vi "GetMeanCurrent.vi"(8 "error in (no error)":errorcluster, 11 "TecellaChannel in":refnum<class "TecellaChannel.lvclass">) -> (0 "error out":errorcluster, 2 "Mean Current (nA)":dbl, 3 "TecellaChannel out":refnum<class "TecellaChannel.lvclass">)   [LabVIEW 2009, in "TecellaChannel.lvclass"]
uses:
  TecellaChannel.lvclass
  TecellaChannel.lvclass/TecellaChannel.ctl
  TecellaClient/TecellaClient.lvclass
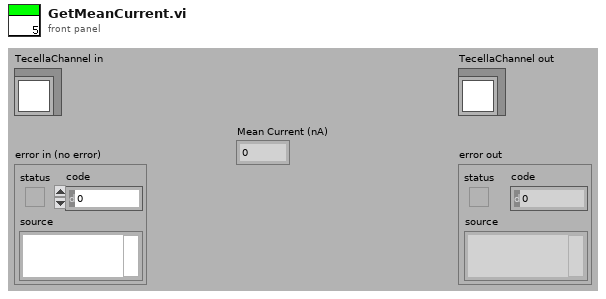
[diagram p1: front panel]
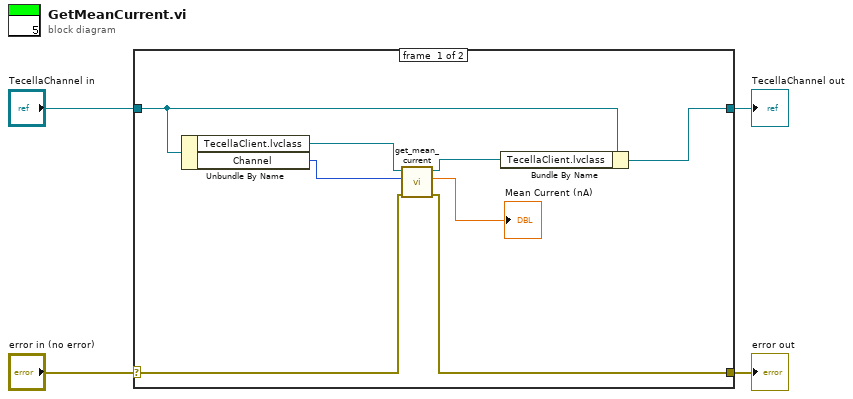
[diagram p0: block diagram]
diagram:
  n1 = case shown="No Error" "error in (no error)" {
    selector: "error in (no error)" -> [w8 w14]
    tunnel: [w7 w14] -> w3
    tunnel: [w11 w13] -> w1
    tunnel: "TecellaChannel in" -> [w12 w13]
    frame #0 {
      n2 = Unbundle By Name(w12) -> ("TecellaClient.lvclass"=w10:refnum<class "TecellaClient.lvclass">, "Channel"=w5:i8)
      n3 = call-dynamic "get_mean_current.vi"("error in (no error)"=w8, "Channel"=w5, "TecellaClient in"=w10) -> ("error out"=w7:errorcluster, "Mean Current (nA)"=→"Mean Current (nA)":dbl, "TecellaClient out"=w9:refnum<class "TecellaClient.lvclass">)  [unwired: 6 in]
      n4 = Bundle By Name(cluster=w12, "TecellaClient.lvclass"=w9) -> (w11:refnum<class "TecellaChannel.lvclass">)
    }
    frame #1 {
    }
  }
  "error out" <- w3
  "TecellaChannel out" <- w1
